vi "Configure Channel (Volt Sqrt).vi"(0 "VISA resource name":refnum<visa-resource-name>, 1 "Scaling":T3={"Floating point position (2)"=2, "Lower Scaling (0)"=0.0, "Upper Scaling (100)"=100.0, "Unit Character (\"\")"=""} {"Upper Scaling (100)" format="%_6g"; "Lower Scaling (0)" format="%_6g"; "Floating point position (2)" min=0 max=5 step=1}, 2 "Low cut":T2 {"Output (0: Zero)" items=["Zero", "Linear"]; "Low-cut (0.0)" min=0.0 max=5.0}, 5 "Channel (0001)":string="0001", 7 "Enable Channel (True)":bool=TRUE, 9 "Range And Span":T1={"Volt Range (4 : 2V)"=4, "Enable Span (False)"=FALSE, "Lower Span (-2.0000)"=-2.0, "Upper Span (2.0000)"=2.0, "Bias (0)"=0.0} {"Upper Span (2.0000)" min=-99999.0 max=99999.0 step=1.0 format="%_5g"; "Lower Span (-2.0000)" min=-99999.0 max=99999.0 step=1.0 format="%_5g"; "Volt Range (4 : 2V)" items=["20mV", "60mV", "200mV", "1V", "2V", "6V", "20V", "50V"]}, 11 "error in (no error)":errorcluster) -> (4 "VISA resource name out":refnum<visa-resource-name>, 6 "Channel":string, 15 "error out":errorcluster)   [LabVIEW 2020, in "Yokogawa GX Series.lvlib"]
doc: "Sets the input range as voltage.\n\nCommand: SRangeAI"
uses:
  <instrlib>/Yokogawa GX Series/Yokogawa GX Series.lvlib
  <instrlib>/Yokogawa GX Series/Private/Volt Range.vi
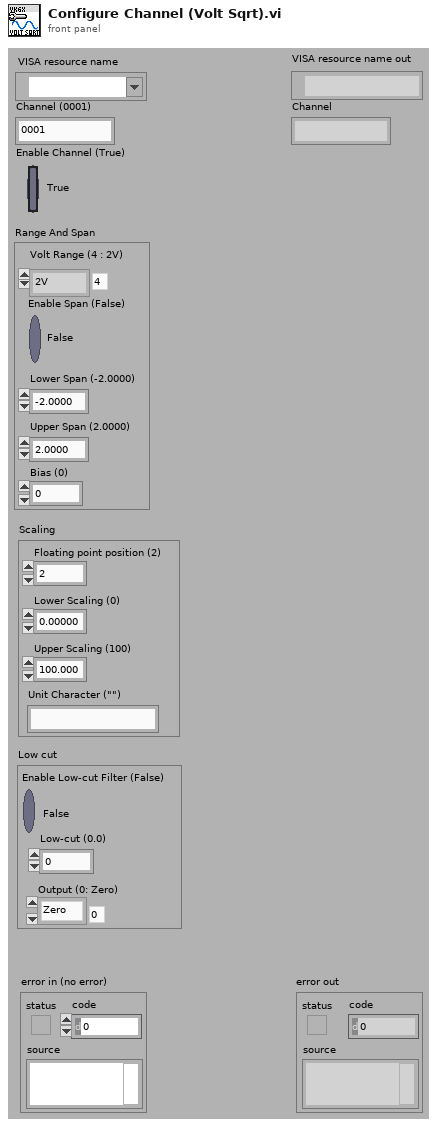
[diagram p1: front panel]
types:
  T1 = cluster{"Volt Range (4 : 2V)":i32, "Enable Span (False)":bool, "Lower Span (-2.0000)":dbl, "Upper Span (2.0000)":dbl, "Bias (0)":dbl}
  T2 = cluster{"Enable Low-cut Filter (False)":bool, "Low-cut (0.0)":dbl, "Output (0: Zero)":u16}
  T3 = cluster{"Floating point position (2)":i32, "Lower Scaling (0)":dbl, "Upper Scaling (100)":dbl, "Unit Character (\"\")":string}
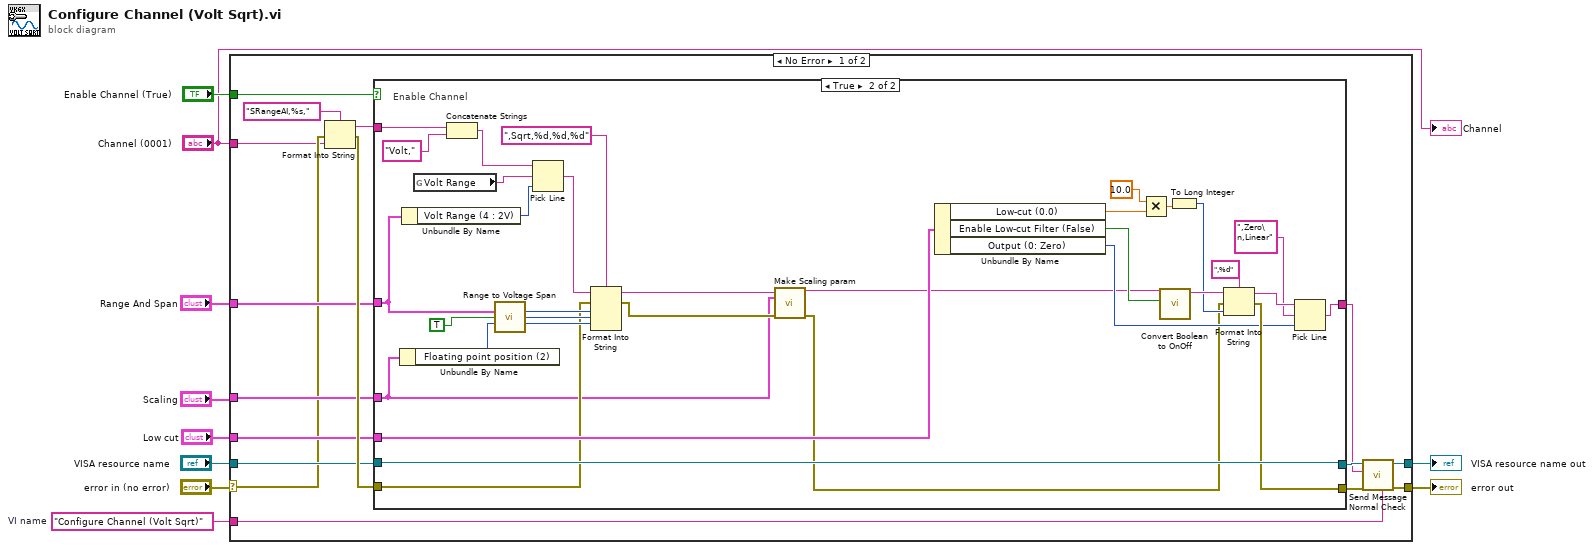
[diagram p0: block diagram]
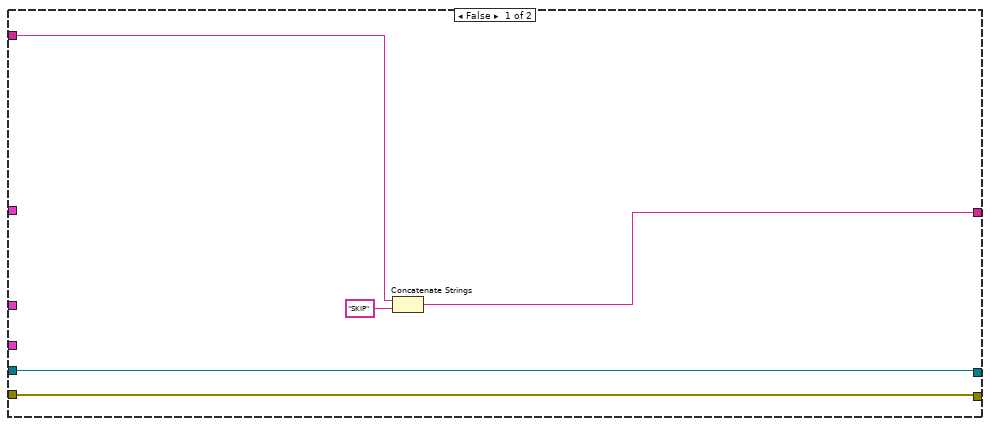
[diagram p2: hidden frame]
diagram:
  w4 = "Configure Channel (Volt Sqrt)"  # VI name
  n1 = case shown="No Error" "error in (no error)" {
    selector: "error in (no error)" -> [w16 w65]
    tunnel: "Enable Channel (True)" -> [w15 _]
    tunnel: "VISA resource name" -> [w23 w66]
    tunnel: "Scaling" -> [w22 _]
    tunnel: "Low cut" -> [w21 _]
    tunnel: [w11 w66] -> w6
    tunnel: [w12 w65] -> w5
    tunnel: w4 -> [w18 _]
    tunnel: "Range And Span" -> [w17 _]
    tunnel: "Channel (0001)" -> [w14 _]
    frame No Error {
      n2 = Format Into String(format string="SRangeAI,%s,", error in=w16, w14) -> (resulting string=w24:string, error out=w25:errorcluster)  [unwired: 1 in]
      n3 = case shown="True" w15 {
        tunnel: w25 -> [w28 w55]
        tunnel: [w28 w54] -> w13
        tunnel: w24 -> [w29 w49]
        tunnel: [w31 w45] -> w19
        tunnel: w23 -> [w27 w56]
        tunnel: [w27 w56] -> w20
        tunnel: w17 -> [_ w53]
        tunnel: w22 -> [_ w35]
        tunnel: w21 -> [_ w57]
        frame False {
          n4 = Concatenate Strings(w29, "SKIP") -> (w31:string)
        }
        frame True {
          # "Enable Channel"
          n5 = Unbundle By Name(w35) -> ("Floating point position (2)"=w40:i32)
          n6 = Unbundle By Name(w53) -> ("Volt Range (4 : 2V)"=w61:i32)
          n7 = global read "Volt Range.vi" "Volt Range"() -> (w32:string)
          n8 = Concatenate Strings(w49, "Volt,") -> (w62:string)
          n9 = call <instrlib>:"Range to Voltage Span.vi"("Range And Span"=w53, "Scaling? (False)"=TRUE, "Floating Point Position (2)"=w40) -> ("Lower Span"=w60:i32, "Upper Span"=w59:i32, "Bias"=w58:i32)  [unwired: 5 in, 5 out]
          n10 = Pick Line(string ("")=w62, multi-line string=w32, line index=w61) -> (output string=w63:string)
          n11 = Format Into String(format string=",Sqrt,%d,%d,%d", initial string=w63, error in=w55, w60, w59, w58) -> (resulting string=w36:string, error out=w38:errorcluster)
          n12 = call <instrlib>:"Make Scaling param.vi"("String (\"\")"=w36, "Scaling"=w35, "error in (no error)"=w38) -> ("String After"=w34:string, "error out"=w37:errorcluster)  [unwired: 11 in]
          n13 = Unbundle By Name(w57) -> ("Low-cut (0.0)"=w43:dbl, "Enable Low-cut Filter (False)"=w51:bool, "Output (0: Zero)"=w50:u16)
          n14 = Multiply(x=10.0, y=w43) -> (x*y=w42:dbl)
          n15 = call <instrlib>:"Convert Boolean to OnOff.vi"("On/Off"=w51, "Initial String (\"\")"=w34) -> ("Resulting String"=w48:string)  [unwired: 9 in]
          n16 = To Long Integer(number=w42) -> (32bit integer=w41:i32)
          n17 = Format Into String(format string=",%d", initial string=w48, error in=w37, w41) -> (resulting string=w47:string, error out=w54:errorcluster)
          n18 = Pick Line(string ("")=w47, multi-line string=",Zero\n,Linear", line index=w50) -> (output string=w45:string)
        }
      }
      n19 = call <instrlib>:"Send Message Normal Check.vi"("Source (\"\")"=w18, "error in (no error)"=w13, "Send Message (\"\")"=w19, "VISA resource name"=w20) -> ("error out"=w12:errorcluster, "VISA resource name out"=w11:refnum<visa-resource-name>)  [unwired: 2 in, 4 out]
    }
    frame Error {
    }
  }
  "error out" <- w5
  "VISA resource name out" <- w6
  "Channel" <- "Channel (0001)"
